vi "GetAxisNames.vi"(8 "error in (no error)":errorcluster, 11 "controller in":refnum<k24>) -> (0 "error out":errorcluster, 2 "axis names":string[](array[string]), 3 "controller out":refnum<k24>)   [LabVIEW 2010]
uses:
  c:/aerotech/controller/5.xx.xxx/A3200/pc/labview/2010/bin/Aerotech.A3200.dll
  bin/Aerotech.A3200.dll
  c:/aerotech/controller/5.xx.xxx/A3200/pc/labview/2010/bin/Aerotech.A3200.LabVIEW.dll
  bin/Aerotech.A3200.LabVIEW.dll
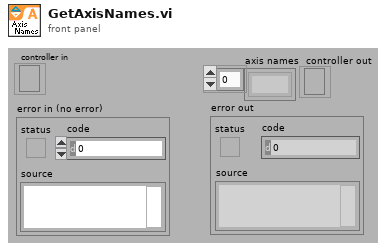
[diagram p1: front panel]
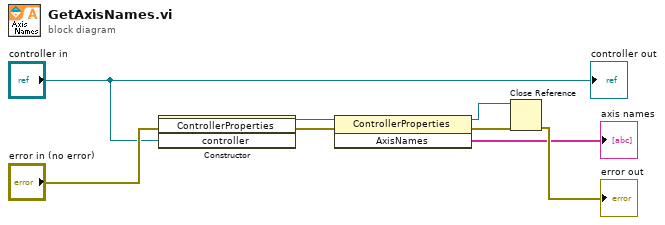
[diagram p0: block diagram]
diagram:
  n1 = constructor class="ControllerProperties"(error in="error in (no error)", "controller"="controller in") -> (reference out=w6:refnum<k24>, error out=w5:errorcluster)  [unwired: 2 in, 2 out]
  n2 = invoke class="ControllerProperties" method="AxisNames"(reference=w6, error in=w5) -> (reference out=w4:refnum<k24>, error out=w3:errorcluster, "AxisNames"=→"axis names":string[])  [unwired: 1 in]
  n3 = Close Reference(reference=w4, error in (no error)=w3) -> (error out=→"error out":errorcluster)
  "controller out" <- "controller in"
